vi "readLuaVariables.vi"() -> ()   [LabVIEW 2009, in "run.lvlib"]
uses:
  run.lvlib
panel:
  out "String":string
  in  "Path":path=path "C:/Users/Administrator/Desktop/Crete/Lua/Sweeping/lvMultiChannels.tsp"
  out "parameters":T1(array[cluster])
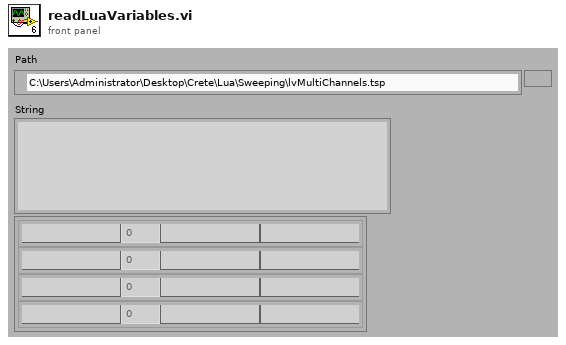
[diagram p1: front panel]
types:
  T1 = cluster{"Name":string, "Value":dbl, "Type":string, "Units":string}[]
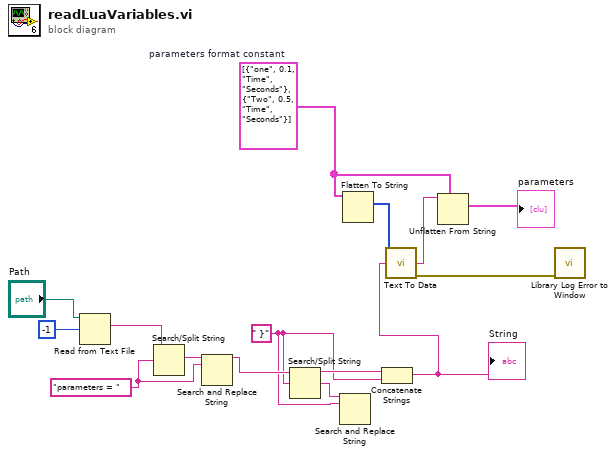
[diagram p0: block diagram]
diagram:
  w2 = " }"
  w6 = "parameters = "
  w11 = T1 [{"Name"="one", "Value"=0.1, "Type"="Time", "Units"="Seconds"}, {"Name"="Two", "Value"=0.5, "Type"="Time", "Units"="Seconds"}]  # parameters format constant
  n1 = Read from Text File(file (use dialog)="Path", count=-1) -> (text=w8:string)  [unwired: 2 in, 3 out]
  n2 = Search/Split String(string=w8, search string/char (-)=w6) -> (match + rest of string=w7:string)  [unwired: 1 in, 2 out]
  n3 = Search and Replace String(input string=w7, search string=w6) -> (result string=w5:string)  [unwired: 6 in, 3 out]
  n4 = Search/Split String(string=w5, search string/char (-)=w2) -> (substring before match=w3:string, match + rest of string=w4:string)  [unwired: 1 in, 1 out]
  n5 = Search and Replace String(input string=w4, search string=w2) -> ()  [unwired: 6 in, 4 out]
  n6 = Flatten To String(anything=w11) -> (type string=w13:i16[])  [unwired: 3 in, 2 out]
  n7 = Concatenate Strings(w3, w2) -> (w1:string)
  "String" <- w1
  n8 = call "Text To Data.vi"("type descriptor"=w13, "text"=w1) -> ("flat data"=w14:string, "error out"=w15:errorcluster)  [unwired: 12 in]
  n9 = Unflatten From String(type=w11, binary string=w14) -> (value=→"parameters":T1)  [unwired: 3 in, 2 out]
  n10 = call "Library Log Error to Window.vi"("error in (no error)"=w15) -> ()  [unwired: 13 in, 2 out]
